vi "RP_Choice_02.vi"(4 "Heading_c":dbl, 5 "vel_veh":dbl, 6 "# of pnt":i32, 7 "WP no_pre":i32, 8 "y_long_c":dbl, 9 "x_lat_c":dbl, 10 "y_long_arr":dbl[](array[numeric]), 11 "x_lat_arr":dbl[](array[numeric])) -> (0 "RP2":T1, 1 "long":dbl[](array[numeric]), 2 "lat":dbl[](array[numeric]), 3 "RP1":T2)   [LabVIEW 2020]
doc: "Reference Point 찾기\n\n주어진 경로상에서 참고할 만한 벡터의 정보 찾기\n--------------RP1-----------------\n인덱스와 헤딩은 속도에 따라 앞에있는 점,\nDist.lane은 현재 떨어진 거리\n--------------RP2-----------------\n현재위치 기준"
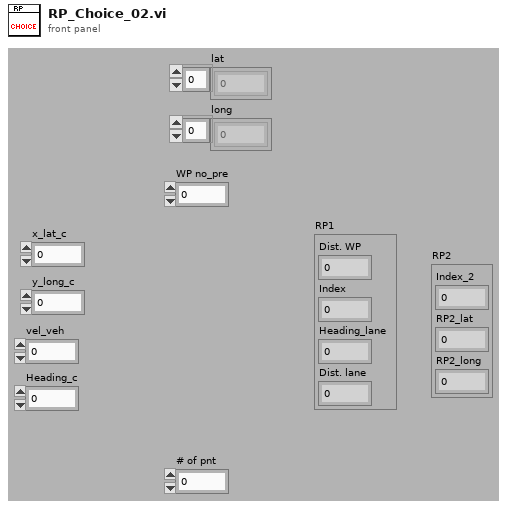
[diagram p1: front panel]
types:
  T1 = cluster{"Index_2":i32, "RP2_lat":dbl, "RP2_long":dbl}
  T2 = cluster{"Dist. WP":dbl, "Index":i32, "Heading_lane":dbl, "Dist. lane":dbl}
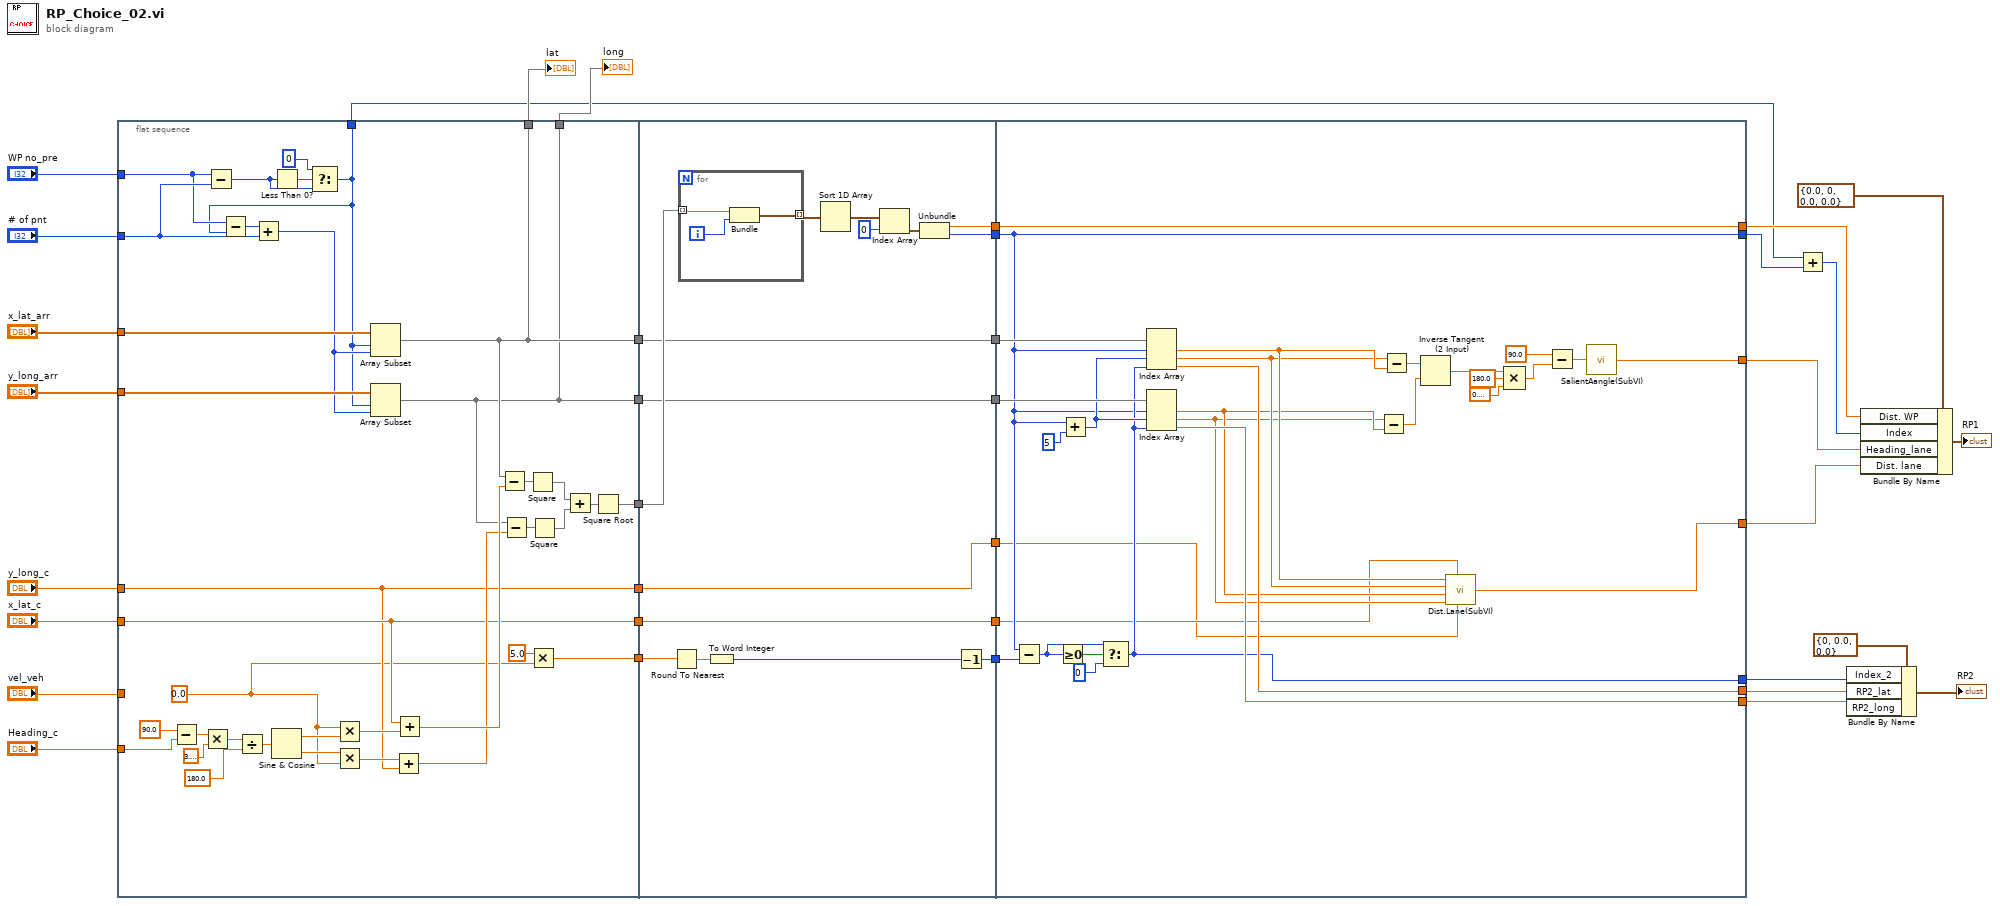
[diagram p0: block diagram]
diagram:
  n1 = flat-sequence {
    tunnel: "WP no_pre" -> [w45]
    tunnel: "# of pnt" -> [w47]
    tunnel: "x_lat_arr" -> [w70]
    tunnel: "y_long_arr" -> [w69]
    tunnel: "x_lat_c" -> [w42]
    tunnel: "y_long_c" -> [w41]
    tunnel: [w63] -> w31
    tunnel: [w40] -> w27
    tunnel: [w39] -> w25
    tunnel: [w42] -> w24
    tunnel: [w41] -> w23
    tunnel: "vel_veh" -> [_]
    tunnel: "Heading_c" -> [w52]
    tunnel: [w43] -> w16
    tunnel: [w40] -> w3
    tunnel: [w39] -> w2
    tunnel: [w38] -> w1
    tunnel: w31 -> [w87]
    tunnel: [w82] -> w30
    tunnel: [w81] -> w29
    tunnel: [w80] -> w28
    tunnel: w27 -> [w80]
    tunnel: [w79] -> w26
    tunnel: w25 -> [w79]
    tunnel: w24 -> [w78]
    tunnel: w23 -> [w77]
    tunnel: [w78] -> w22
    tunnel: [w77] -> w21
    tunnel: w16 -> [w76]
    tunnel: [w74] -> w15
    tunnel: w30 -> [w103]
    tunnel: w29 -> [w98]
    tunnel: w28 -> [w119]
    tunnel: w26 -> [w118]
    tunnel: w22 -> [w92]
    tunnel: w21 -> [w91]
    tunnel: [w93] -> w11
    tunnel: [w98] -> w20
    tunnel: w15 -> [w108]
    tunnel: [w103] -> w14
    tunnel: [w102] -> w12
    tunnel: [w100] -> w7
    tunnel: [w101] -> w6
    tunnel: [w99] -> w8
    frame #0 {
      w37 = 0.0 ("y")
      n2 = Subtract(x=90.0, y=w52) -> (x-y=w57:dbl)
      n3 = Multiply(x=w57, y=3.141592653589793) -> (x*y=w55:dbl)
      n4 = Subtract(x=w45, y=w47) -> (x-y=w49:i32)
      n5 = Divide(x=w55, y=180.0) -> (x/y=w53:dbl)
      n6 = Less Than 0?(x=w49) -> (x < 0?=w72:bool)
      n7 = Sine & Cosine(0:w53) -> (1:w62:dbl, 2:w61:dbl)
      n8 = Select(t=0, s=w72, f=w49) -> (s? t:f=w38:i32)
      n9 = Subtract(x=w45, y=w38) -> (x-y=w48:i32)
      n10 = Add(x=w48, y=w47) -> (x+y=w46:i32)
      n11 = Multiply(x=w37, y=w62) -> (x*y=w60:dbl)
      n12 = Multiply(x=w61, y=w37) -> (x*y=w59:dbl)
      n13 = Array Subset(array=w70, index=w38, length=w46) -> (w40:dbl[])
      n14 = Array Subset(array=w69, index=w38, length=w46) -> (w39:dbl[])
      n15 = Add(x=w59, y=w41) -> (x+y=w50:dbl)
      n16 = Add(x=w42, y=w60) -> (x+y=w51:dbl)
      n17 = Subtract(x=w40, y=w51) -> (x-y=w68:dbl[])
      n18 = Subtract(x=w39, y=w50) -> (x-y=w67:dbl[])
      n19 = Square(x=w68) -> (x^2=w66:dbl[])
      n20 = Multiply(x=5.0, y=w37) -> (x*y=w43:dbl)
      n21 = Square(x=w67) -> (x^2=w65:dbl[])
      n22 = Add(x=w66, y=w65) -> (x+y=w64:dbl[])
      n23 = Square Root(x=w64) -> (sqrt(x)=w63:dbl[])
    }
    frame #1 {
      n24 = Round To Nearest(number=w76) -> (nearest integer value=w75:dbl)
      n25 = for {
        tunnel: w87 -> [w90] mode=indexing
        tunnel: [w89] -> w86 mode=indexing
        i -> [w88]
        n26 = Bundle(w90, w88) -> (w89:cluster{dbl, i32})  [unwired: 1 in]
      }
      n27 = To Word Integer(number=w75) -> (16bit integer=w73:i16)
      n28 = Sort 1D Array(array=w86) -> (sorted array=w85:cluster{dbl, i32}[])
      n29 = Index Array(array=w85, index=0) -> (element=w83:cluster{dbl, i32})
      n30 = Unbundle(w83) -> (w82:dbl, w81:i32)
      n31 = Decrement(x=w73) -> (x-1=w74:i16)
    }
    frame #2 {
      n32 = Subtract(x=w98, y=w108) -> (x-y=w106:i32)
      n33 = Greater Or Equal To 0?(x=w106) -> (x >= 0?=w107:bool)
      n34 = Add(x=w98, y=5) -> (x+y=w104:i32)
      n35 = Select(t=w106, s=w107, f=0) -> (s? t:f=w99:i32)
      n36 = Index Array(array=w119, index #1=w98, index #2=w104, index #3=w99) -> (element #1=w97:dbl, element #2=w96:dbl, element #3=w100:dbl)
      n37 = Index Array(array=w118, index #1=w98, index #2=w104, index #3=w99) -> (element #1=w95:dbl, element #2=w94:dbl, element #3=w101:dbl)
      n38 = Subtract(x=w94, y=w95) -> (x-y=w117:dbl)
      n39 = Subtract(x=w96, y=w97) -> (x-y=w116:dbl)
      n40 = Inverse Tangent (2 Input)(1:w117, 2:w116) -> (0:w111:dbl)
      n41 = call "Dist.Lane(SubVI).vi"("x0"=w91, "y0"=w92, "x2"=w94, "x1"=w95, "y2"=w96, "y1"=w97) -> ("Dist.Lane"=w93:dbl)
      n42 = Compound Arithmetic op=MULTIPLY(w111, 180.0 ("value"), 0.3183098861837907) -> (w112:dbl)
      n43 = Subtract(x=90.0, y=w112) -> (x-y=w110:dbl)
      n44 = call "SalientAangle(SubVI).vi"("angle"=w110) -> ("salient angle"=w102:dbl)
    }
  }
  n45 = Add(x=w1, y=w20) -> (x+y=w13:i32)
  n46 = Bundle By Name(cluster=T1 {"Index_2"=0, "RP2_lat"=0.0, "RP2_long"=0.0}, "Index_2"=w8, "RP2_lat"=w7, "RP2_long"=w6) -> (→"RP2":T1)
  n47 = Bundle By Name(cluster=T2 {"Dist. WP"=0.0, "Index"=0, "Heading_lane"=0.0, "Dist. lane"=0.0}, "Dist. WP"=w14, "Index"=w13, "Heading_lane"=w12, "Dist. lane"=w11) -> (→"RP1":T2)
  "lat" <- w3
  "long" <- w2
